vi "temperature_controller_write.vi"(1 "Value":string, 2 "Command":string, 3 "delay before read (ms)":u32=75, 4 "VISA resource name":refnum<visa-resource-name>="COM1") -> (0 "Read Buffer":string)   [LabVIEW 2011]
uses:
  <vilib>/Instr/_visa.llb/VISA Configure Serial Port (Instr).vi
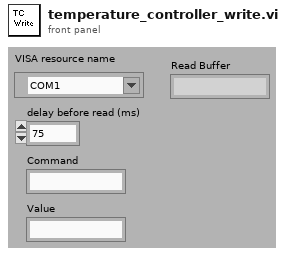
[diagram p1: front panel]
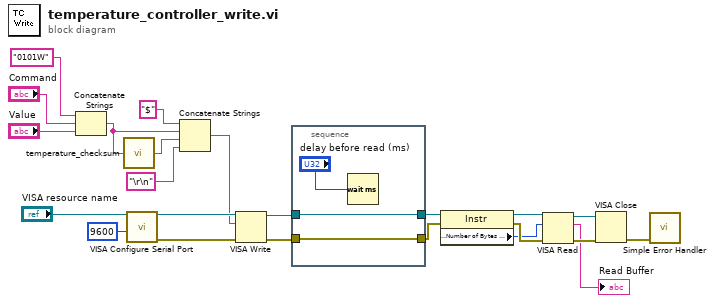
[diagram p0: block diagram]
diagram:
  n1 = Concatenate Strings("0101W" ("write buffer"), "Command", "Value") -> (w10:string)
  n2 = call "temperature_checksum.vi"("Input string"=w10) -> ("Checksum"=w9:string)
  n3 = call-poly "VISA Configure Serial Port"("VISA resource name"="VISA resource name", "baud rate (9600)"=u32 9600) -> ("VISA resource name out"=w19:refnum<visa-resource-name>, "error out"=w18:errorcluster)  [unwired: 4 in, 8 out]
  n4 = Concatenate Strings("$" ("string"), w10, w9, "\r\n" ("string")) -> (w5:string)
  n5 = VISA Write(VISA resource name=w19, write buffer=w5, error in (no error)=w18) -> (VISA resource name out=w20:refnum<visa-resource-name>, error out=w21:errorcluster)  [unwired: 1 out]
  n6 = stacked-sequence {
    tunnel: w21 -> [w26]
    tunnel: [w26] -> w17
    tunnel: w20 -> [w25]
    tunnel: [w25] -> w16
    frame #0 {
      n7 = Wait (ms)(milliseconds to wait="delay before read (ms)") -> ()  [unwired: 1 out]
    }
  }
  n8 = property class="Instr"(reference=w16, error in=w17) -> (reference out=w15:refnum<visa-resource-name>, error out=w14:errorcluster, "Serial Settings:Number of Bytes at Serial Port"=w13:u32)
  n9 = VISA Read(VISA resource name=w15, byte count=w13, error in (no error)=w14) -> (VISA resource name out=w12:refnum<visa-resource-name>, read buffer=→"Read Buffer":string, error out=w11:errorcluster)  [unwired: 1 out]
  n10 = VISA Close(VISA resource name=w12, error in (no error)=w11) -> (error out=w22:errorcluster)
  n11 = call <vilib>:"Simple Error Handler.vi"("error in (no error)"=w22) -> ()  [unwired: 1 in, 8 out]
